vi "ISEG_HVBoard.ProcCases.vi"(0 "i ref in":refnum<vi>, 1 "selector":string, 2 "Data":T1, 3 "call cluster":T2={"Object"="", "Selector"="", "CallType"=enum."synchronous", "Async Object"="", "Async Selector"="", "Data Descriptor"="", "Data"=[], "Error #"=0, "Expire"=0}, 5 "error in (no error)":errorcluster) -> (14 "i ref out":refnum<vi>, 17 "answer cluster":T2={"Object"="", "Selector"="", "CallType"=enum."synchronous", "Async Object"="", "Async Selector"="", "Data Descriptor"="", "Data"=[], "Error #"=0, "Expire"=0}, 19 "error out":errorcluster)   [LabVIEW 2014, in "ISEG_HVBoard.lvlib"]
doc: "This method is called by a process from within the default case in the event loop. The methods of a class that are linked to events will be called from THIS method. Add your code here."
uses:
  ISEG_HVBoard.lvlib
  CSCore/CSSystem/CoreDefs/CoreDefs.call_type.ctl
  CSCore/BaseProcess/BaseProcess.descriptor string definition.ctl
  CSCore/CSSystem/CoreDefs/CoreDefs.rawDataType.ctl
  CSCore/CSApplicationBaseClasses/DeviceBase/DeviceBase.deviceState.ctl
  CSCore/CSSystem/CoreLib/CoreLib.string 2 byte array.vi
  CSCore/CSSystem/CoreLib/CoreLib.byte array 2 double.vi
  CSCore/CSSystem/CoreLib/CoreLib.double 2 byte array.vi
  CSCore/CSSystem/CoreLib/CoreLib.short 2 byte array.vi
  CSCore/CSSystem/CoreLib/CoreLib.byte array 2 short.vi
  CSCore/CSApplicationBaseClasses/DeviceBase/DeviceBase.lvlib
  CSCore/CSSystem/CoreLib/CoreLib.lvlib
  CSCore/BaseProcess/BaseProcess.lvlib
  CSCore/CAEObj/CAEObj.lvlib
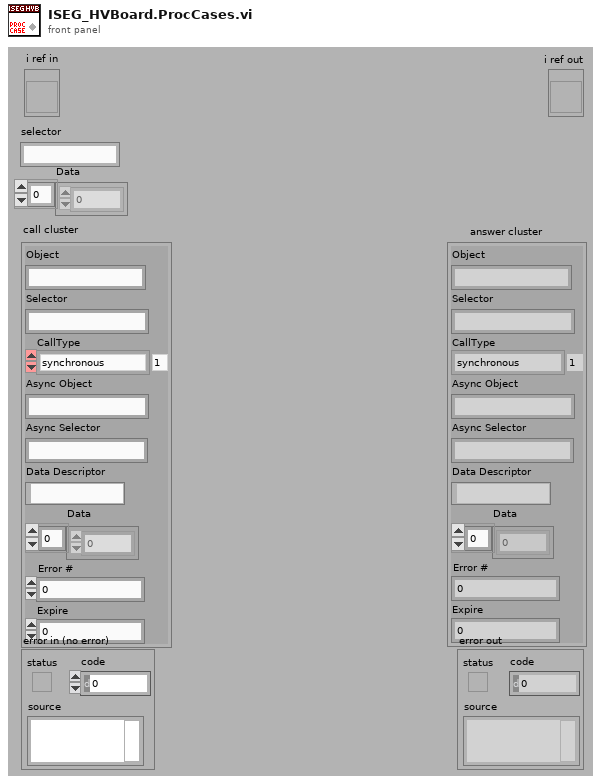
[diagram p1: front panel]
types:
  T1 = typedef "CoreDefs.rawDataType.ctl" = i8[]
  T2 = typedef "CoreDefs.call_type.ctl" = cluster{"Object":string, "Selector":string, "CallType":enum16{"simple", "synchronous", "asynchronous"}, "Async Object":string, "Async Selector":string, "Data Descriptor":T3, "Data":T1, "Error #":i32, "Expire":u32}
  T3 = typedef "BaseProcess.lvlib/BaseProcess.descriptor string definition.ctl" = string
  T4 = typedef "ISEG_HVBoard.lvlib/ISEG_HVBoard.i attribute.ctl" = cluster{"System Name":string, "Board ID":i32, "Prefix":string, "NrOfCh":cluster{"NrOfCh":i16, "DIM Status":T5}, "Status":cluster{"Status":i16, "DIM Status":T5}, "HardwareVLimit":cluster{"HVMax":dbl, "DIM Status":T5}, "BoardTemp":cluster{"Temp":dbl, "DIM Status":T5}, " Emcy":cluster{"Emcy":bool, "DIM Status":T5}}
  T5 = typedef "ISEG_HVBoard.lvlib/ISEG_HVBoard.DIM Status.ctl" = cluster{"no link":bool, "quality":i32, "Time Stamp":timestamp}
  T6 = typedef "DeviceBase.lvlib/DeviceBase.i attribute.ctl" = cluster{"deviceState":i32, "deviceStateID":i32, "deviceID":string, "deviceIDID":i32, "advancedGUIClass":string, "advancedGUIClassID":i32}
  T7 = typedef "DeviceBase.lvlib/DeviceBase.deviceState.ctl" = i16
  T8 = typedef "BaseProcess.lvlib/BaseProcess.i attribute.ctl" = cluster{"EventStatus":string, "EventError":i32, "PresetEvtWatchD":i32, "PresetPdcWatchD":i32, "EventTimeout":i32, "PeriodicInterval":i32, "Interface":string[], "Address":string[], "Special":string[], "PeriodicError":i32, "PeriodicStatus":string, "SuperProc":string, "Descriptors":T9[], "CaseRef":refnum<vi>, "PdcRef":refnum<vi>, "Thread Ref":refnum<vi>, "eventErrorID":i32, "eventStatusID":i32, "periodicErrorID":i32, "periodicStatusID":i32, "pdcCtrID":i32}
  T9 = typedef "BaseProcess.lvlib/BaseProcess.descriptor definition.ctl" = cluster{"selector":string, "descriptor":T3}
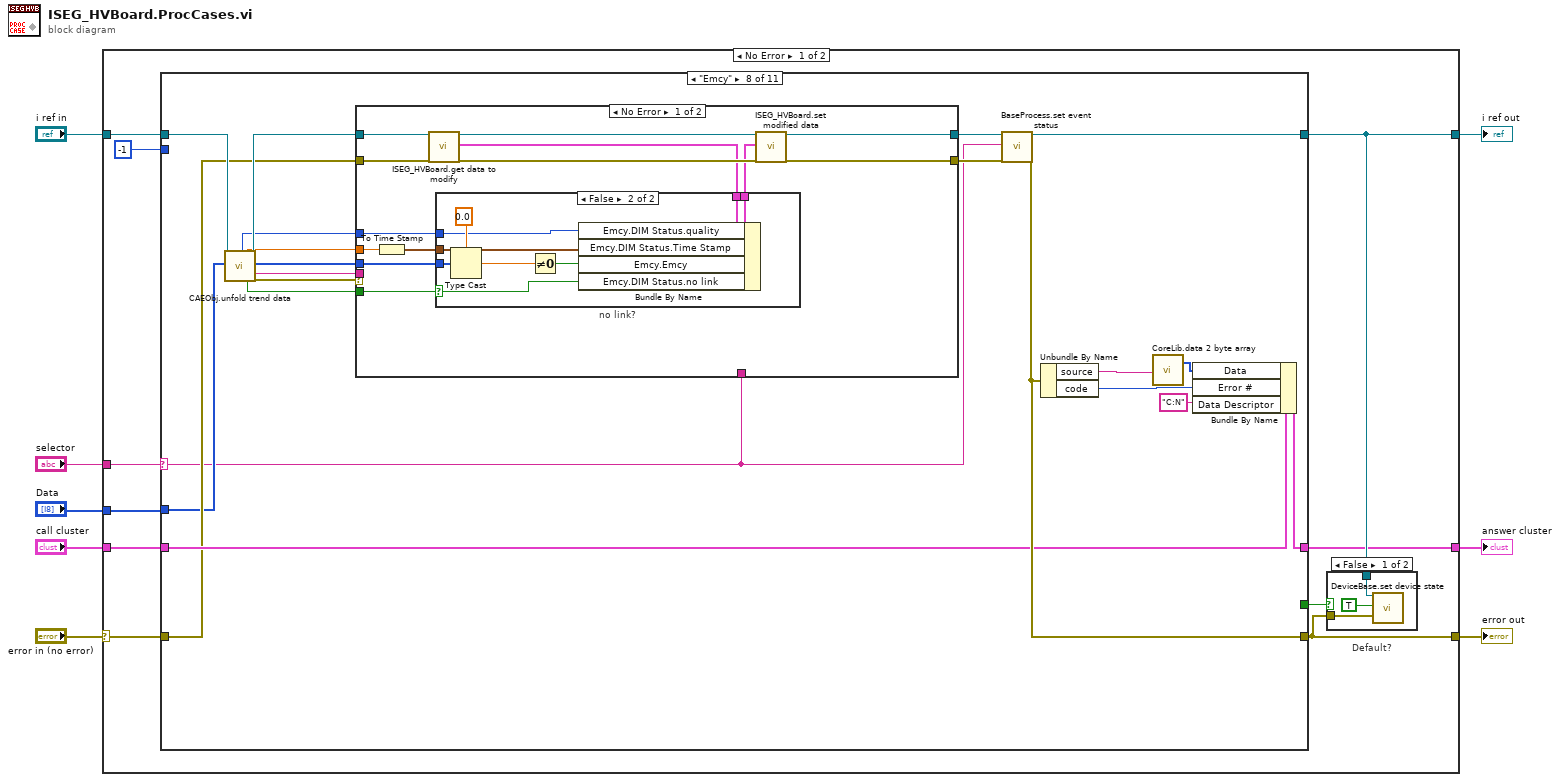
[diagram p0: block diagram]
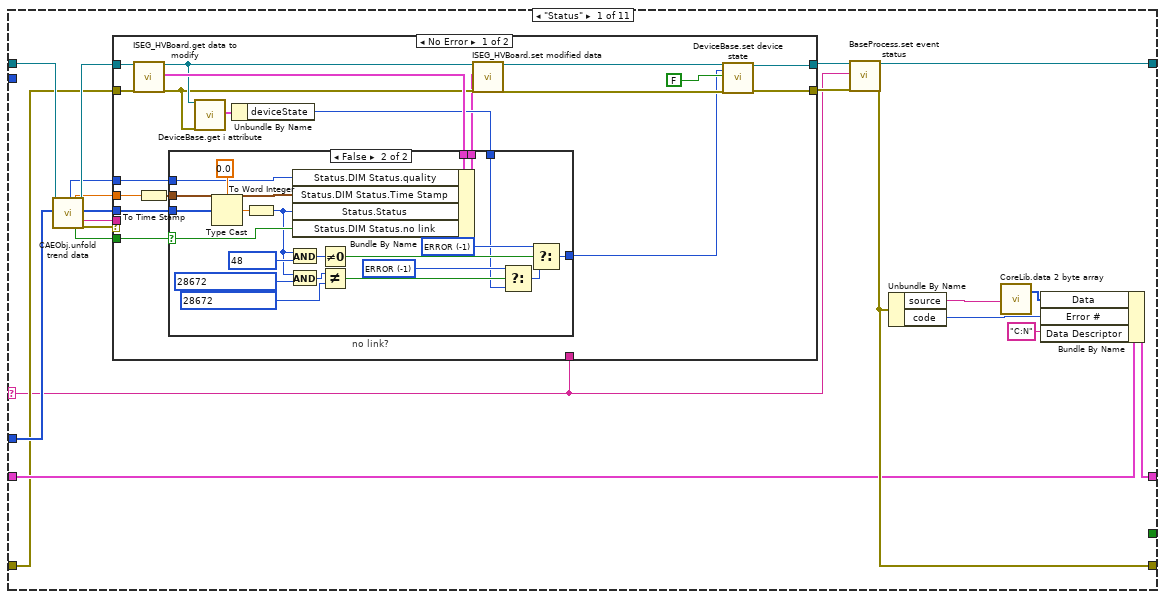
[diagram p3: hidden frame]
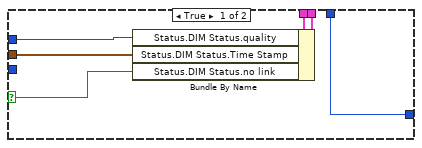
[diagram p4: hidden frame]
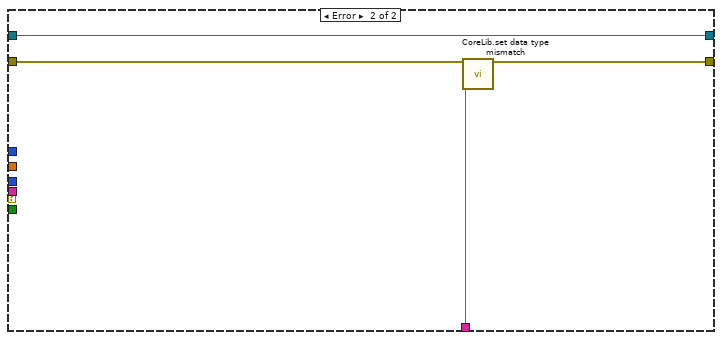
[diagram p5: hidden frame]
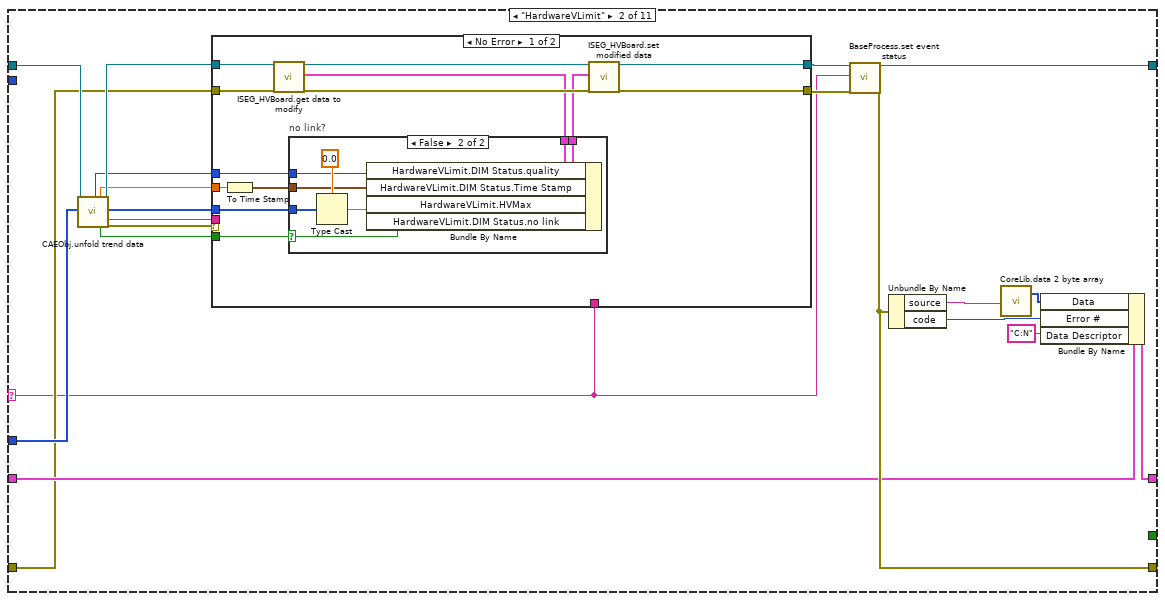
[diagram p6: hidden frame]
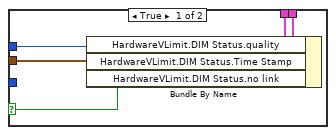
[diagram p7: hidden frame]
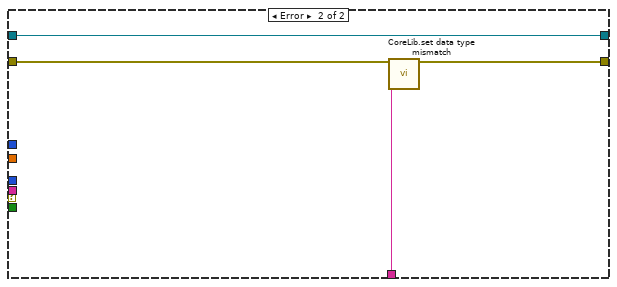
[diagram p8: hidden frame]
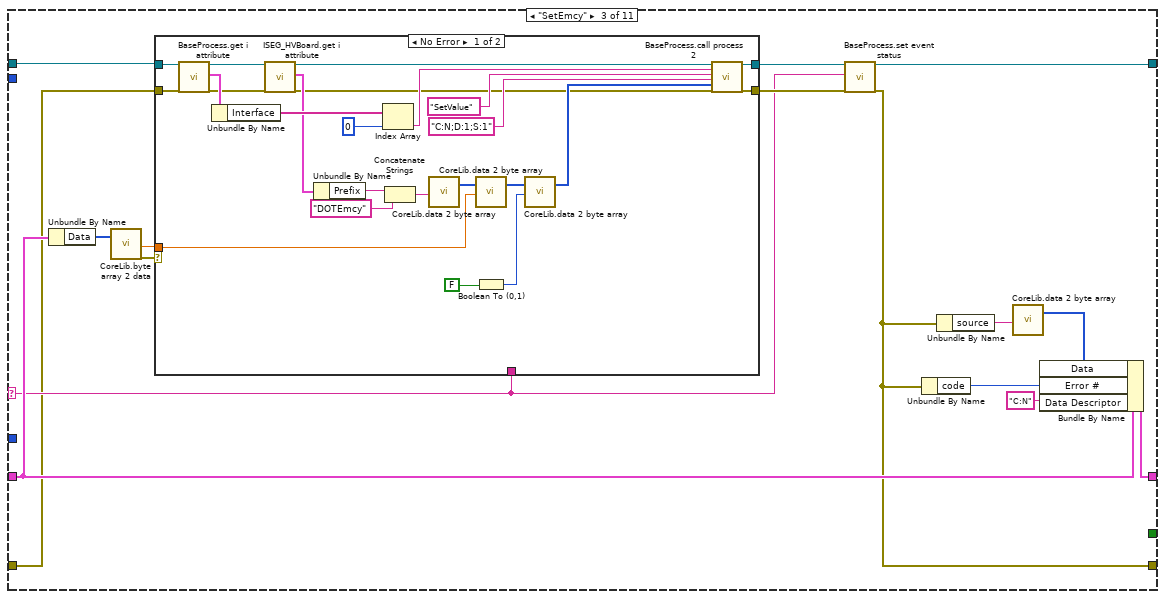
[diagram p9: hidden frame]
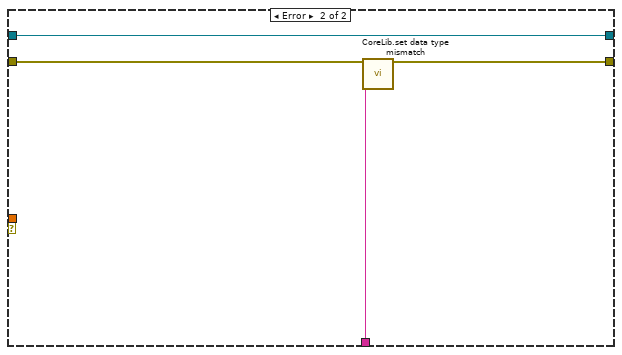
[diagram p10: hidden frame]
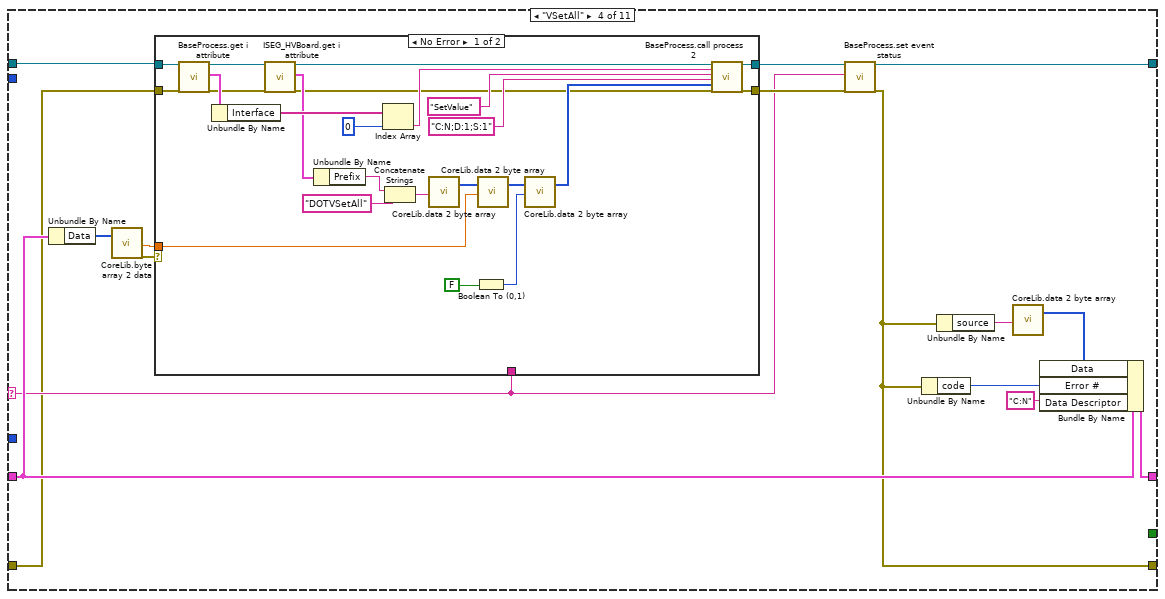
[diagram p11: hidden frame]
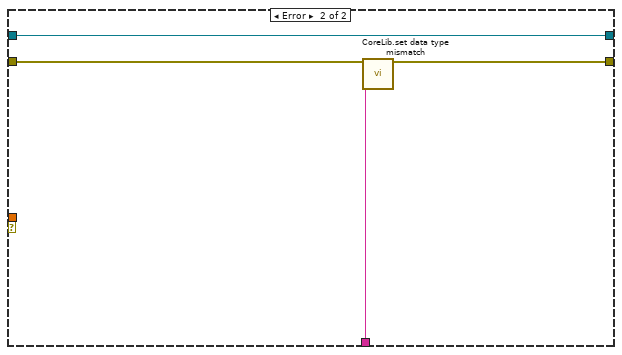
[diagram p12: hidden frame]
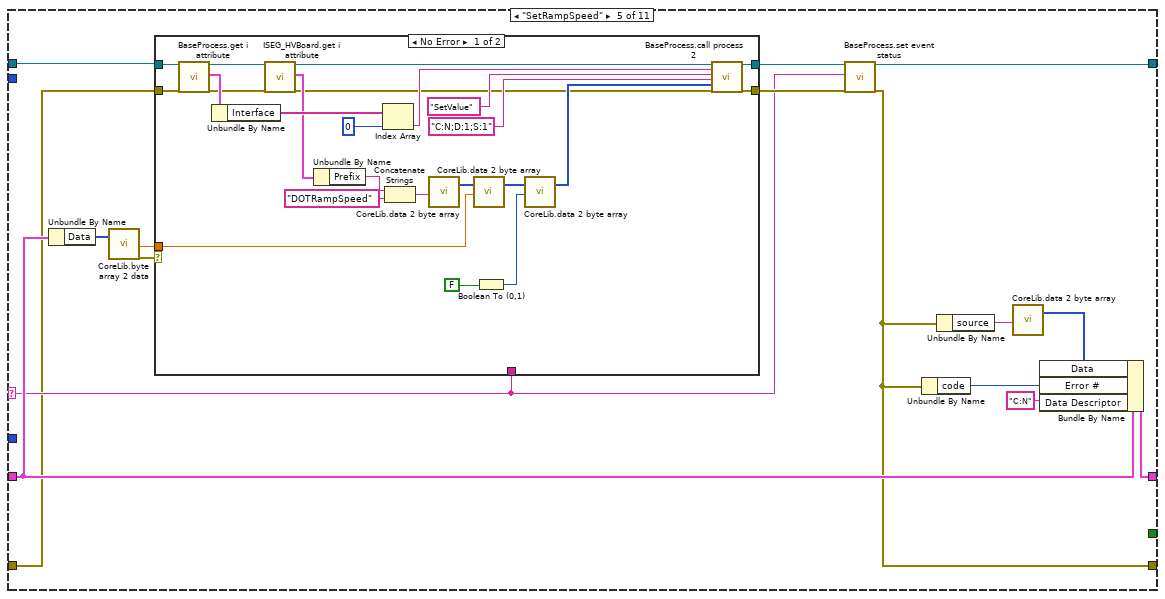
[diagram p13: hidden frame]
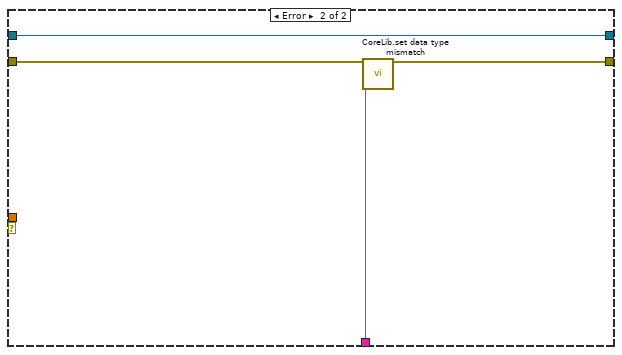
[diagram p14: hidden frame]
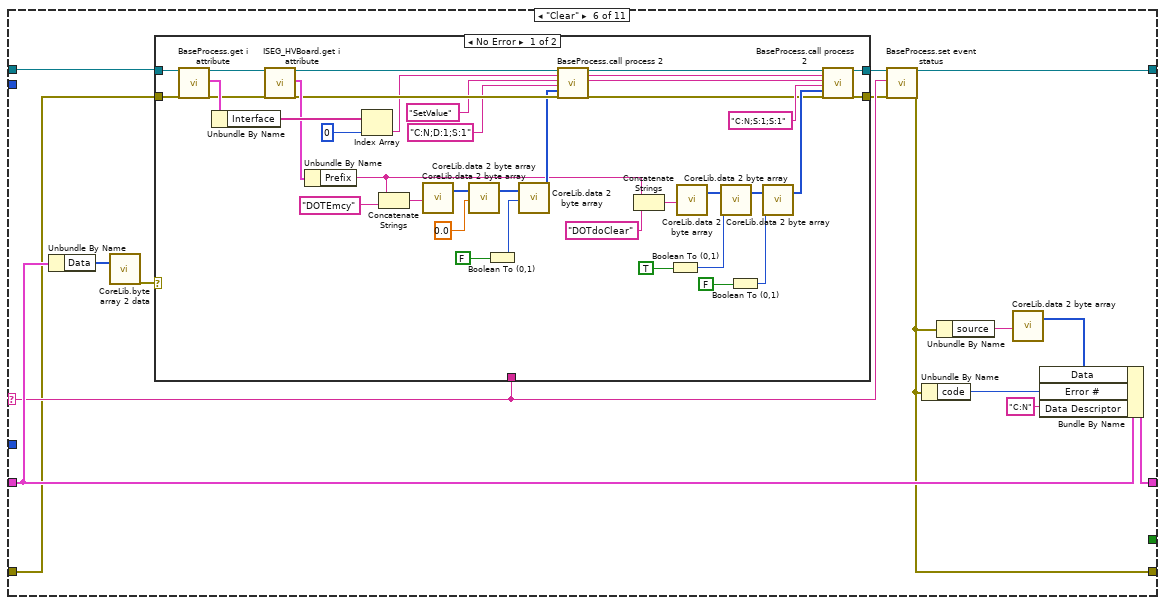
[diagram p15: hidden frame]
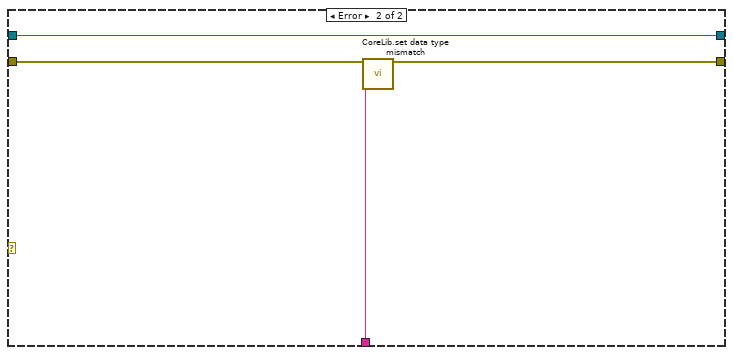
[diagram p16: hidden frame]
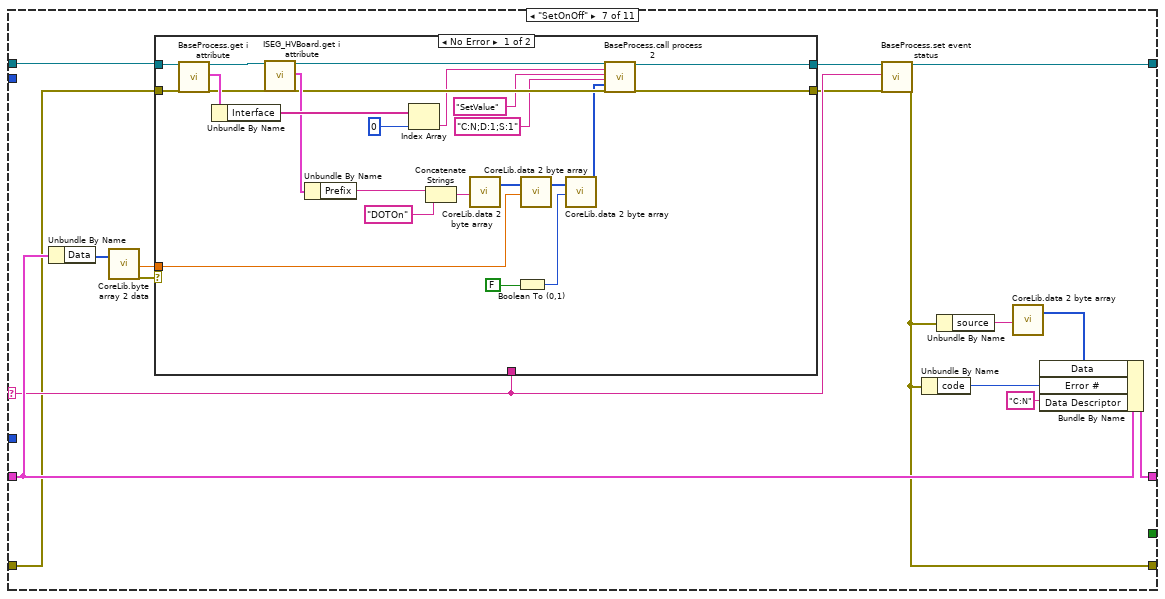
[diagram p17: hidden frame]
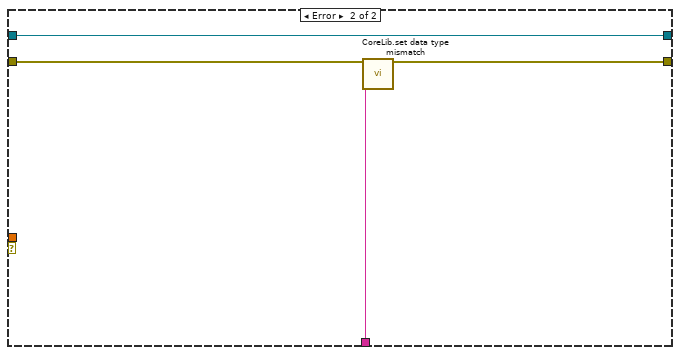
[diagram p18: hidden frame]
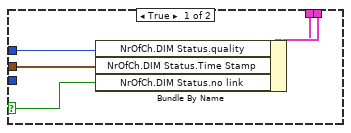
[diagram p19: hidden frame]
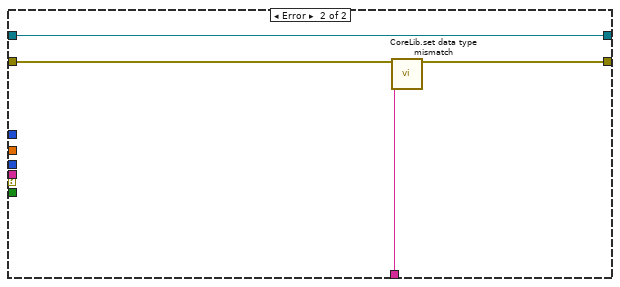
[diagram p20: hidden frame]
diagram:
  n1 = case shown="No Error" "error in (no error)" {
    selector: "error in (no error)" -> [w13 w538]
    tunnel: "selector" -> [w16 _]
    tunnel: [w10 w539] -> w7
    tunnel: "Data" -> [w15 _]
    tunnel: "call cluster" -> [w14 w539]
    tunnel: "i ref in" -> [w18 w540]
    tunnel: [w11 w540] -> w3
    tunnel: [w9 w538] -> w2
    frame No Error {
      n2 = case shown="\"Emcy\"" w16 {
        selector: w16 -> [w22 w93 w150 w194 w238 w282 w338 w375 w429 w479 w532]
        tunnel: w15 -> [w26 w97 _ _ _ _ _ w376 w430 w483 _]
        tunnel: w18 -> [w27 w98 w153 w197 w241 w285 w341 w380 w432 w484 w531]
        tunnel: [w37 w107 w152 w196 w240 w284 w340 w389 w441 w493 w537] -> w11
        tunnel: w14 -> [w36 w106 w151 w195 w239 w283 w339 w388 w440 w492 w533]
        tunnel: [w35 w108 w147 w191 w235 w279 w335 w390 w442 w494 w534] -> w10
        tunnel: w13 -> [w23 w96 w148 w192 w236 w280 w336 w377 w431 w482 w536]
        tunnel: [w38 w109 w149 w193 w237 w281 w337 w391 w443 w495 w535] -> w9
        tunnel: [_ _ _ _ _ _ _ _ _ _ TRUE] -> w12
        tunnel: -1 -> [_ _ _ _ _ _ _ _ _ _ _]
        frame "Status" {
          n3 = call "CAEObj.unfold trend data.vi"("i ref in"=w27, "raw trend data"=w26) -> ("quality"=w31:i32, "timeStamp"=w30:dbl, "no link"=w28:bool, "i ref out"=w34:refnum<vi>, "data"=w33:i8[], "typeDescriptor"=w32:string, "error out"=w29:errorcluster)  [unwired: 9 in, 2 out]
          n4 = case shown="No Error" w29 {
            tunnel: [w47 w92] -> w25
            tunnel: w34 -> [w61 w92]
            tunnel: w23 -> [w60 w91]
            tunnel: [w46 w90] -> w24
            tunnel: w22 -> [_ w89]
            tunnel: w33 -> [w59 _]
            tunnel: w32 -> [_ _]
            tunnel: w31 -> [w57 _]
            tunnel: w30 -> [w55 _]
            tunnel: w28 -> [w54 _]
            frame No Error {
              n5 = call "ISEG_HVBoard.get data to modify.vi"("i ref in"=w61, "error in (no error)"=w60) -> ("i ref out"=w52:refnum<vi>, "i attribute"=w58:T4, "error out"=w51:errorcluster)  [unwired: 14 in, 1 out]
              n6 = To Time Stamp(1:w55) -> (0:w56:timestamp)
              n7 = call "DeviceBase.get i attribute.vi"("i ref in"=w52, "error in (no error)"=w51) -> ("i attribute"=w53:T6)  [unwired: 15 in, 2 out]
              n8 = Unbundle By Name(w53) -> ("deviceState"=w44:i32)
              n9 = case "no link?" shown="False" w54 {
                selector: w54 -> [w63 w81]
                tunnel: [w67 w88] -> w43
                tunnel: w59 -> [_ w87]
                tunnel: w58 -> [w66 w86]
                tunnel: w57 -> [w65 w83]
                tunnel: w56 -> [w64 w82]
                tunnel: [w62 w77] -> w45
                tunnel: w44 -> [w62 w70]
                frame True {
                  n10 = Bundle By Name(cluster=w66, "Status.DIM Status.quality"=w65, "Status.DIM Status.Time Stamp"=w64, "Status.DIM Status.no link"=w63) -> (w67:T4)
                }
                frame False {
                  w72 = T7 -1 items=["ERROR"=-1, "OK"=0, "NOT_OK"=1] ("deviceState")
                  w80 = T7 -1 items=["ERROR"=-1, "OK"=0, "NOT_OK"=1] ("deviceState")
                  n11 = Type Cast(type=0.0, x=w87) -> (*(type *) &x=w85:dbl)
                  n12 = To Word Integer(number=w85) -> (16bit integer=w75:i16)
                  n13 = And(x=w75, y=i16 48) -> (x .and. y?=w79:i16)
                  n14 = And(x=w75, y=i16 28672) -> (x .and. y?=w69:i16)
                  n15 = Bundle By Name(cluster=w86, "Status.DIM Status.quality"=w83, "Status.DIM Status.Time Stamp"=w82, "Status.Status"=w75, "Status.DIM Status.no link"=w81) -> (w88:T4)
                  n16 = Not Equal To 0?(x=w79) -> (x != 0?=w78:bool)
                  n17 = Not Equal?(x=w69, y=i16 28672) -> (x != y?=w73:bool)
                  n18 = Select(t=w72, s=w73, f=w70) -> (s? t:f=w71:i32)
                  n19 = Select(t=w80, s=w78, f=w71) -> (s? t:f=w77:i32)
                }
              }
              n20 = call "ISEG_HVBoard.set modified data.vi"("i ref in"=w52, "i attribute"=w43, "error in (no error)"=w51) -> ("i ref out"=w48:refnum<vi>, "error out"=w49:errorcluster)  [unwired: 15 in]
              n21 = call "DeviceBase.set device state.vi"("i ref in"=w48, "deviceState"=w45, "implicit"=FALSE, "error in (no error)"=w49) -> ("i ref out"=w47:refnum<vi>, "error out"=w46:errorcluster)  [unwired: 13 in, 1 out]
            }
            frame Error {
              n22 = call "CoreLib.set data type mismatch.vi"("error in (no error)"=w91, "error source"=w89) -> ("error out"=w90:errorcluster)  [unwired: 17 in]
            }
          }
          n23 = call "BaseProcess.set event status.vi"("i ref in"=w25, "EventStatus"=w22, "error in (no error)"=w24) -> ("i ref out"=w37:refnum<vi>, "error out"=w38:errorcluster)  [unwired: 14 in, 1 out]
          n24 = Unbundle By Name(w38) -> ("source"=w39:string, "code"=w42:i32)
          n25 = call-poly "CoreLib.data 2 byte array.vi"("string"=w39) -> ("byteArray out"=w41:T1)  [unwired: 18 in]
          n26 = Bundle By Name(cluster=w36, "Data"=w41, "Error #"=w42, "Data Descriptor"="C:N") -> (w35:T2)
        }
        frame "HardwareVLimit" {
          n27 = call "CAEObj.unfold trend data.vi"("i ref in"=w98, "raw trend data"=w97) -> ("quality"=w102:i32, "timeStamp"=w101:dbl, "no link"=w99:bool, "i ref out"=w105:refnum<vi>, "data"=w104:i8[], "typeDescriptor"=w103:string, "error out"=w100:errorcluster)  [unwired: 9 in, 2 out]
          n28 = case shown="No Error" w100 {
            tunnel: [w120 w143] -> w94
            tunnel: w105 -> [w126 w143]
            tunnel: w96 -> [w125 w142]
            tunnel: [w119 w141] -> w95
            tunnel: w93 -> [_ w140]
            tunnel: w104 -> [w121 _]
            tunnel: w103 -> [_ _]
            tunnel: w102 -> [w117 _]
            tunnel: w101 -> [w115 _]
            tunnel: w99 -> [w114 _]
            frame No Error {
              n29 = To Time Stamp(1:w115) -> (0:w116:timestamp)
              n30 = call "ISEG_HVBoard.get data to modify.vi"("i ref in"=w126, "error in (no error)"=w125) -> ("i ref out"=w124:refnum<vi>, "i attribute"=w118:T4, "error out"=w123:errorcluster)  [unwired: 14 in, 1 out]
              n31 = case "no link?" shown="False" w114 {
                selector: w114 -> [w127 w133]
                tunnel: [w131 w139] -> w122
                tunnel: w121 -> [_ w138]
                tunnel: w118 -> [w130 w136]
                tunnel: w117 -> [w129 w135]
                tunnel: w116 -> [w128 w134]
                frame True {
                  n32 = Bundle By Name(cluster=w130, "HardwareVLimit.DIM Status.quality"=w129, "HardwareVLimit.DIM Status.Time Stamp"=w128, "HardwareVLimit.DIM Status.no link"=w127) -> (w131:T4)
                }
                frame False {
                  n33 = Type Cast(type=0.0, x=w138) -> (*(type *) &x=w132:dbl)
                  n34 = Bundle By Name(cluster=w136, "HardwareVLimit.DIM Status.quality"=w135, "HardwareVLimit.DIM Status.Time Stamp"=w134, "HardwareVLimit.HVMax"=w132, "HardwareVLimit.DIM Status.no link"=w133) -> (w139:T4)
                }
              }
              n35 = call "ISEG_HVBoard.set modified data.vi"("i ref in"=w124, "i attribute"=w122, "error in (no error)"=w123) -> ("i ref out"=w120:refnum<vi>, "error out"=w119:errorcluster)  [unwired: 15 in]
            }
            frame Error {
              n36 = call "CoreLib.set data type mismatch.vi"("error in (no error)"=w142, "error source"=w140) -> ("error out"=w141:errorcluster)  [unwired: 17 in]
            }
          }
          n37 = call "BaseProcess.set event status.vi"("i ref in"=w94, "EventStatus"=w93, "error in (no error)"=w95) -> ("i ref out"=w107:refnum<vi>, "error out"=w109:errorcluster)  [unwired: 14 in, 1 out]
          n38 = Unbundle By Name(w109) -> ("source"=w110:string, "code"=w113:i32)
          n39 = call-poly "CoreLib.data 2 byte array.vi"("string"=w110) -> ("byteArray out"=w112:T1)  [unwired: 18 in]
          n40 = Bundle By Name(cluster=w106, "Data"=w112, "Error #"=w113, "Data Descriptor"="C:N") -> (w108:T2)
        }
        frame "SetEmcy" {
          n41 = Unbundle By Name(w151) -> ("Data"=w144:T1)
          n42 = call-poly "CoreLib.byte array 2 data.vi"("byteArray"=w144) -> ("d64"=w146:dbl, "error out"=w145:errorcluster)  [unwired: 16 in, 1 out]
          n43 = case shown="No Error" w145 {
            tunnel: [w183 w187] -> w157
            tunnel: w153 -> [w169 w187]
            tunnel: w148 -> [w181 w186]
            tunnel: [w182 w185] -> w156
            tunnel: w150 -> [_ w184]
            tunnel: w146 -> [w160 _]
            frame No Error {
              n44 = call "BaseProcess.get i attribute.vi"("i ref in"=w169, "error in (no error)"=w181) -> ("i ref out"=w164:refnum<vi>, "i attribute"=w180:T8, "error out"=w166:errorcluster)  [unwired: 15 in]
              n45 = Unbundle By Name(w180) -> ("Interface"=w179:string[])
              n46 = call "ISEG_HVBoard.get i attribute.vi"("i ref in"=w164, "error in (no error)"=w166) -> ("i ref out"=w163:refnum<vi>, "i attribute"=w168:T4, "error out"=w165:errorcluster)  [unwired: 15 in]
              n47 = Unbundle By Name(w168) -> ("Prefix"=w167:string)
              n48 = Index Array(array=w179, index=0) -> (element=w177:string)
              n49 = Concatenate Strings(w167, "DOTEmcy" ("string")) -> (w171:string)
              n50 = call-poly "CoreLib.data 2 byte array.vi"("string"=w171) -> ("byteArray out"=w162:T1)  [unwired: 18 in]
              n51 = call-poly "CoreLib.data 2 byte array.vi"("byteArray"=w162, "f64"=w160) -> ("byteArray out"=w161:T1)  [unwired: 17 in]
              n52 = Boolean To (0,1)(Boolean=FALSE) -> (0, 1=w173:i16)
              n53 = call-poly "CoreLib.data 2 byte array.vi"("byteArray"=w161, "i16"=w173) -> ("byteArray out"=w172:T1)  [unwired: 17 in]
              n54 = call "BaseProcess.call process 2.vi"("i ref in"=w163, "Object"=w177, "Selector"="SetValue", "Data Descriptor"="C:N;D:1;S:1", "Data"=w172, "error in (no error)"=w165) -> ("i ref out"=w183:refnum<vi>, "error out"=w182:errorcluster)  [unwired: 12 in]
            }
            frame Error {
              n55 = call "CoreLib.set data type mismatch.vi"("error in (no error)"=w186, "error source"=w184) -> ("error out"=w185:errorcluster)  [unwired: 17 in]
            }
          }
          n56 = call "BaseProcess.set event status.vi"("i ref in"=w157, "EventStatus"=w150, "error in (no error)"=w156) -> ("i ref out"=w152:refnum<vi>, "error out"=w149:errorcluster)  [unwired: 14 in, 1 out]
          n57 = Unbundle By Name(w149) -> ("code"=w159:i32)
          n58 = Unbundle By Name(w149) -> ("source"=w154:string)
          n59 = call-poly "CoreLib.data 2 byte array.vi"("string"=w154) -> ("byteArray out"=w158:T1)  [unwired: 18 in]
          n60 = Bundle By Name(cluster=w151, "Data"=w158, "Error #"=w159, "Data Descriptor"="C:N") -> (w147:T2)
        }
        frame "VSetAll" {
          n61 = Unbundle By Name(w195) -> ("Data"=w188:T1)
          n62 = call-poly "CoreLib.byte array 2 data.vi"("byteArray"=w188) -> ("d64"=w190:dbl, "error out"=w189:errorcluster)  [unwired: 16 in, 1 out]
          n63 = case shown="No Error" w189 {
            tunnel: [w227 w231] -> w201
            tunnel: w197 -> [w213 w231]
            tunnel: w192 -> [w225 w230]
            tunnel: [w226 w229] -> w200
            tunnel: w194 -> [_ w228]
            tunnel: w190 -> [w204 _]
            frame No Error {
              n64 = call "BaseProcess.get i attribute.vi"("i ref in"=w213, "error in (no error)"=w225) -> ("i ref out"=w208:refnum<vi>, "i attribute"=w224:T8, "error out"=w210:errorcluster)  [unwired: 15 in]
              n65 = Unbundle By Name(w224) -> ("Interface"=w223:string[])
              n66 = call "ISEG_HVBoard.get i attribute.vi"("i ref in"=w208, "error in (no error)"=w210) -> ("i ref out"=w207:refnum<vi>, "i attribute"=w212:T4, "error out"=w209:errorcluster)  [unwired: 15 in]
              n67 = Unbundle By Name(w212) -> ("Prefix"=w211:string)
              n68 = Index Array(array=w223, index=0) -> (element=w221:string)
              n69 = Concatenate Strings(w211, "DOTVSetAll" ("string")) -> (w215:string)
              n70 = call-poly "CoreLib.data 2 byte array.vi"("string"=w215) -> ("byteArray out"=w205:T1)  [unwired: 18 in]
              n71 = Boolean To (0,1)(Boolean=FALSE) -> (0, 1=w217:i16)
              n72 = call-poly "CoreLib.data 2 byte array.vi"("byteArray"=w205, "f64"=w204) -> ("byteArray out"=w206:T1)  [unwired: 17 in]
              n73 = call-poly "CoreLib.data 2 byte array.vi"("byteArray"=w206, "i16"=w217) -> ("byteArray out"=w216:T1)  [unwired: 17 in]
              n74 = call "BaseProcess.call process 2.vi"("i ref in"=w207, "Object"=w221, "Selector"="SetValue", "Data Descriptor"="C:N;D:1;S:1", "Data"=w216, "error in (no error)"=w209) -> ("i ref out"=w227:refnum<vi>, "error out"=w226:errorcluster)  [unwired: 12 in]
            }
            frame Error {
              n75 = call "CoreLib.set data type mismatch.vi"("error in (no error)"=w230, "error source"=w228) -> ("error out"=w229:errorcluster)  [unwired: 17 in]
            }
          }
          n76 = call "BaseProcess.set event status.vi"("i ref in"=w201, "EventStatus"=w194, "error in (no error)"=w200) -> ("i ref out"=w196:refnum<vi>, "error out"=w193:errorcluster)  [unwired: 14 in, 1 out]
          n77 = Unbundle By Name(w193) -> ("code"=w203:i32)
          n78 = Unbundle By Name(w193) -> ("source"=w198:string)
          n79 = call-poly "CoreLib.data 2 byte array.vi"("string"=w198) -> ("byteArray out"=w202:T1)  [unwired: 18 in]
          n80 = Bundle By Name(cluster=w195, "Data"=w202, "Error #"=w203, "Data Descriptor"="C:N") -> (w191:T2)
        }
        frame "SetRampSpeed" {
          n81 = Unbundle By Name(w239) -> ("Data"=w232:T1)
          n82 = call-poly "CoreLib.byte array 2 data.vi"("byteArray"=w232) -> ("d64"=w234:dbl, "error out"=w233:errorcluster)  [unwired: 16 in, 1 out]
          n83 = case shown="No Error" w233 {
            tunnel: [w271 w275] -> w245
            tunnel: w241 -> [w258 w275]
            tunnel: w236 -> [w269 w274]
            tunnel: [w270 w273] -> w244
            tunnel: w238 -> [_ w272]
            tunnel: w234 -> [w248 _]
            frame No Error {
              n84 = call "BaseProcess.get i attribute.vi"("i ref in"=w258, "error in (no error)"=w269) -> ("i ref out"=w253:refnum<vi>, "i attribute"=w268:T8, "error out"=w255:errorcluster)  [unwired: 15 in]
              n85 = Unbundle By Name(w268) -> ("Interface"=w267:string[])
              n86 = call "ISEG_HVBoard.get i attribute.vi"("i ref in"=w253, "error in (no error)"=w255) -> ("i ref out"=w252:refnum<vi>, "i attribute"=w257:T4, "error out"=w254:errorcluster)  [unwired: 15 in]
              n87 = Unbundle By Name(w257) -> ("Prefix"=w256:string)
              n88 = Index Array(array=w267, index=0) -> (element=w265:string)
              n89 = Concatenate Strings(w256, "DOTRampSpeed" ("string")) -> (w259:string)
              n90 = call-poly "CoreLib.data 2 byte array.vi"("string"=w259) -> ("byteArray out"=w250:T1)  [unwired: 18 in]
              n91 = call-poly "CoreLib.data 2 byte array.vi"("byteArray"=w250, "f64"=w248) -> ("byteArray out"=w249:T1)  [unwired: 17 in]
              n92 = Boolean To (0,1)(Boolean=FALSE) -> (0, 1=w261:i16)
              n93 = call-poly "CoreLib.data 2 byte array.vi"("byteArray"=w249, "i16"=w261) -> ("byteArray out"=w260:T1)  [unwired: 17 in]
              n94 = call "BaseProcess.call process 2.vi"("i ref in"=w252, "Object"=w265, "Selector"="SetValue", "Data Descriptor"="C:N;D:1;S:1", "Data"=w260, "error in (no error)"=w254) -> ("i ref out"=w271:refnum<vi>, "error out"=w270:errorcluster)  [unwired: 12 in]
            }
            frame Error {
              n95 = call "CoreLib.set data type mismatch.vi"("error in (no error)"=w274, "error source"=w272) -> ("error out"=w273:errorcluster)  [unwired: 17 in]
            }
          }
          n96 = call "BaseProcess.set event status.vi"("i ref in"=w245, "EventStatus"=w238, "error in (no error)"=w244) -> ("i ref out"=w240:refnum<vi>, "error out"=w237:errorcluster)  [unwired: 14 in, 1 out]
          n97 = Unbundle By Name(w237) -> ("code"=w247:i32)
          n98 = Unbundle By Name(w237) -> ("source"=w242:string)
          n99 = call-poly "CoreLib.data 2 byte array.vi"("string"=w242) -> ("byteArray out"=w246:T1)  [unwired: 18 in]
          n100 = Bundle By Name(cluster=w239, "Data"=w246, "Error #"=w247, "Data Descriptor"="C:N") -> (w235:T2)
        }
        frame "Clear" {
          n101 = Unbundle By Name(w283) -> ("Data"=w276:T1)
          n102 = call-poly "CoreLib.byte array 2 data.vi"("byteArray"=w276) -> ("error out"=w277:errorcluster)  [unwired: 16 in, 2 out]
          n103 = case shown="No Error" w277 {
            tunnel: [w298 w330] -> w288
            tunnel: w285 -> [w323 w330]
            tunnel: w280 -> [w326 w329]
            tunnel: w282 -> [_ w328]
            tunnel: [w297 w327] -> w278
            frame No Error {
              w294 = "SetValue" ("Selector")
              n104 = call "BaseProcess.get i attribute.vi"("i ref in"=w323, "error in (no error)"=w326) -> ("i ref out"=w319:refnum<vi>, "i attribute"=w325:T8, "error out"=w321:errorcluster)  [unwired: 15 in]
              n105 = Unbundle By Name(w325) -> ("Interface"=w324:string[])
              n106 = call "ISEG_HVBoard.get i attribute.vi"("i ref in"=w319, "error in (no error)"=w321) -> ("i ref out"=w318:refnum<vi>, "i attribute"=w322:T4, "error out"=w320:errorcluster)  [unwired: 15 in]
              n107 = Unbundle By Name(w322) -> ("Prefix"=w296:string)
              n108 = Index Array(array=w324, index=0) -> (element=w295:string)
              n109 = Concatenate Strings(w296, "DOTEmcy" ("string")) -> (w312:string)
              n110 = call-poly "CoreLib.data 2 byte array.vi"("string"=w312) -> ("byteArray out"=w293:T1)  [unwired: 18 in]
              n111 = call-poly "CoreLib.data 2 byte array.vi"("byteArray"=w293, "f64"=0.0) -> ("byteArray out"=w292:T1)  [unwired: 17 in]
              n112 = Boolean To (0,1)(Boolean=FALSE) -> (0, 1=w314:i16)
              n113 = call-poly "CoreLib.data 2 byte array.vi"("byteArray"=w292, "i16"=w314) -> ("byteArray out"=w313:T1)  [unwired: 17 in]
              n114 = call "BaseProcess.call process 2.vi"("i ref in"=w318, "Object"=w295, "Selector"=w294, "Data Descriptor"="C:N;D:1;S:1", "Data"=w313, "error in (no error)"=w320) -> ("i ref out"=w300:refnum<vi>, "error out"=w299:errorcluster)  [unwired: 12 in]
              n115 = Concatenate Strings(w296, "DOTdoClear" ("string")) -> (w308:string)
              n116 = Boolean To (0,1)(Boolean=TRUE) -> (0, 1=w305:i16)
              n117 = call-poly "CoreLib.data 2 byte array.vi"("string"=w308) -> ("byteArray out"=w304:T1)  [unwired: 18 in]
              n118 = call-poly "CoreLib.data 2 byte array.vi"("byteArray"=w304, "i16"=w305) -> ("byteArray out"=w303:T1)  [unwired: 17 in]
              n119 = Boolean To (0,1)(Boolean=FALSE) -> (0, 1=w309:i16)
              n120 = call-poly "CoreLib.data 2 byte array.vi"("byteArray"=w303, "i16"=w309) -> ("byteArray out"=w301:T1)  [unwired: 17 in]
              n121 = call "BaseProcess.call process 2.vi"("i ref in"=w300, "Object"=w295, "Selector"=w294, "Data Descriptor"="C:N;S:1;S:1", "Data"=w301, "error in (no error)"=w299) -> ("i ref out"=w298:refnum<vi>, "error out"=w297:errorcluster)  [unwired: 12 in]
            }
            frame Error {
              n122 = call "CoreLib.set data type mismatch.vi"("error in (no error)"=w329, "error source"=w328) -> ("error out"=w327:errorcluster)  [unwired: 17 in]
            }
          }
          n123 = call "BaseProcess.set event status.vi"("i ref in"=w288, "EventStatus"=w282, "error in (no error)"=w278) -> ("i ref out"=w284:refnum<vi>, "error out"=w281:errorcluster)  [unwired: 14 in, 1 out]
          n124 = Unbundle By Name(w281) -> ("code"=w290:i32)
          n125 = Unbundle By Name(w281) -> ("source"=w286:string)
          n126 = call-poly "CoreLib.data 2 byte array.vi"("string"=w286) -> ("byteArray out"=w289:T1)  [unwired: 18 in]
          n127 = Bundle By Name(cluster=w283, "Data"=w289, "Error #"=w290, "Data Descriptor"="C:N") -> (w279:T2)
        }
        frame "SetOnOff" {
          n128 = Unbundle By Name(w339) -> ("Data"=w331:T1)
          n129 = call-poly "CoreLib.byte array 2 data.vi"("byteArray"=w331) -> ("d64"=w333:dbl, "error out"=w332:errorcluster)  [unwired: 16 in, 1 out]
          n130 = case shown="No Error" w332 {
            tunnel: [w359 w374] -> w344
            tunnel: w341 -> [w367 w374]
            tunnel: w336 -> [w370 w373]
            tunnel: w338 -> [_ w372]
            tunnel: [w360 w371] -> w334
            tunnel: w333 -> [w347 _]
            frame No Error {
              n131 = call "BaseProcess.get i attribute.vi"("i ref in"=w367, "error in (no error)"=w370) -> ("i ref out"=w363:refnum<vi>, "i attribute"=w369:T8, "error out"=w365:errorcluster)  [unwired: 15 in]
              n132 = Unbundle By Name(w369) -> ("Interface"=w368:string[])
              n133 = call "ISEG_HVBoard.get i attribute.vi"("i ref in"=w363, "error in (no error)"=w365) -> ("i ref out"=w362:refnum<vi>, "i attribute"=w366:T4, "error out"=w364:errorcluster)  [unwired: 15 in]
              n134 = Unbundle By Name(w366) -> ("Prefix"=w361:string)
              n135 = Index Array(array=w368, index=0) -> (element=w351:string)
              n136 = Concatenate Strings(w361, "DOTOn" ("string")) -> (w353:string)
              n137 = call-poly "CoreLib.data 2 byte array.vi"("string"=w353) -> ("byteArray out"=w348:T1)  [unwired: 18 in]
              n138 = Boolean To (0,1)(Boolean=FALSE) -> (0, 1=w355:i16)
              n139 = call-poly "CoreLib.data 2 byte array.vi"("byteArray"=w348, "f64"=w347) -> ("byteArray out"=w349:T1)  [unwired: 17 in]
              n140 = call-poly "CoreLib.data 2 byte array.vi"("byteArray"=w349, "i16"=w355) -> ("byteArray out"=w354:T1)  [unwired: 17 in]
              n141 = call "BaseProcess.call process 2.vi"("i ref in"=w362, "Object"=w351, "Selector"="SetValue", "Data Descriptor"="C:N;D:1;S:1", "Data"=w354, "error in (no error)"=w364) -> ("i ref out"=w359:refnum<vi>, "error out"=w360:errorcluster)  [unwired: 12 in]
            }
            frame Error {
              n142 = call "CoreLib.set data type mismatch.vi"("error in (no error)"=w373, "error source"=w372) -> ("error out"=w371:errorcluster)  [unwired: 17 in]
            }
          }
          n143 = call "BaseProcess.set event status.vi"("i ref in"=w344, "EventStatus"=w338, "error in (no error)"=w334) -> ("i ref out"=w340:refnum<vi>, "error out"=w337:errorcluster)  [unwired: 14 in, 1 out]
          n144 = Unbundle By Name(w337) -> ("code"=w346:i32)
          n145 = Unbundle By Name(w337) -> ("source"=w342:string)
          n146 = call-poly "CoreLib.data 2 byte array.vi"("string"=w342) -> ("byteArray out"=w345:T1)  [unwired: 18 in]
          n147 = Bundle By Name(cluster=w339, "Data"=w345, "Error #"=w346, "Data Descriptor"="C:N") -> (w335:T2)
        }
        frame "Emcy" {
          n148 = call "CAEObj.unfold trend data.vi"("i ref in"=w380, "raw trend data"=w376) -> ("quality"=w383:i32, "timeStamp"=w382:dbl, "no link"=w381:bool, "i ref out"=w387:refnum<vi>, "data"=w386:i8[], "typeDescriptor"=w385:string, "error out"=w384:errorcluster)  [unwired: 9 in, 2 out]
          n149 = case shown="No Error" w384 {
            tunnel: [w401 w426] -> w379
            tunnel: w387 -> [w408 w426]
            tunnel: w377 -> [w407 w425]
            tunnel: [w400 w424] -> w378
            tunnel: w375 -> [_ w423]
            tunnel: w386 -> [w403 _]
            tunnel: w385 -> [_ _]
            tunnel: w383 -> [w399 _]
            tunnel: w382 -> [w398 _]
            tunnel: w381 -> [w396 _]
            frame No Error {
              n150 = To Time Stamp(1:w398) -> (0:w397:timestamp)
              n151 = call "ISEG_HVBoard.get data to modify.vi"("i ref in"=w408, "error in (no error)"=w407) -> ("i ref out"=w406:refnum<vi>, "i attribute"=w402:T4, "error out"=w405:errorcluster)  [unwired: 14 in, 1 out]
              n152 = case "no link?" shown="False" w396 {
                selector: w396 -> [w409 w416]
                tunnel: [w413 w422] -> w404
                tunnel: w403 -> [_ w421]
                tunnel: w402 -> [w412 w420]
                tunnel: w399 -> [w411 w418]
                tunnel: w397 -> [w410 w417]
                frame True {
                  n153 = Bundle By Name(cluster=w412, "NrOfCh.DIM Status.quality"=w411, "NrOfCh.DIM Status.Time Stamp"=w410, "NrOfCh.DIM Status.no link"=w409) -> (w413:T4)
                }
                frame False {
                  n154 = Type Cast(type=0.0, x=w421) -> (*(type *) &x=w414:dbl)
                  n155 = Not Equal To 0?(x=w414) -> (x != 0?=w415:bool)
                  n156 = Bundle By Name(cluster=w420, "Emcy.DIM Status.quality"=w418, "Emcy.DIM Status.Time Stamp"=w417, "Emcy.Emcy"=w415, "Emcy.DIM Status.no link"=w416) -> (w422:T4)
                }
              }
              n157 = call "ISEG_HVBoard.set modified data.vi"("i ref in"=w406, "i attribute"=w404, "error in (no error)"=w405) -> ("i ref out"=w401:refnum<vi>, "error out"=w400:errorcluster)  [unwired: 15 in]
            }
            frame Error {
              n158 = call "CoreLib.set data type mismatch.vi"("error in (no error)"=w425, "error source"=w423) -> ("error out"=w424:errorcluster)  [unwired: 17 in]
            }
          }
          n159 = call "BaseProcess.set event status.vi"("i ref in"=w379, "EventStatus"=w375, "error in (no error)"=w378) -> ("i ref out"=w389:refnum<vi>, "error out"=w391:errorcluster)  [unwired: 14 in, 1 out]
          n160 = Unbundle By Name(w391) -> ("source"=w392:string, "code"=w395:i32)
          n161 = call-poly "CoreLib.data 2 byte array.vi"("string"=w392) -> ("byteArray out"=w394:T1)  [unwired: 18 in]
          n162 = Bundle By Name(cluster=w388, "Data"=w394, "Error #"=w395, "Data Descriptor"="C:N") -> (w390:T2)
        }
        frame "NrOfCh" {
          n163 = call "CAEObj.unfold trend data.vi"("i ref in"=w432, "raw trend data"=w430) -> ("quality"=w435:i32, "timeStamp"=w434:dbl, "no link"=w433:bool, "i ref out"=w439:refnum<vi>, "data"=w438:i8[], "typeDescriptor"=w437:string, "error out"=w436:errorcluster)  [unwired: 9 in, 2 out]
          n164 = case shown="No Error" w436 {
            tunnel: [w453 w478] -> w427
            tunnel: w439 -> [w460 w478]
            tunnel: w431 -> [w459 w477]
            tunnel: [w452 w476] -> w428
            tunnel: w429 -> [_ w475]
            tunnel: w438 -> [w455 _]
            tunnel: w437 -> [_ _]
            tunnel: w435 -> [w451 _]
            tunnel: w434 -> [w450 _]
            tunnel: w433 -> [w448 _]
            frame No Error {
              n165 = To Time Stamp(1:w450) -> (0:w449:timestamp)
              n166 = call "ISEG_HVBoard.get data to modify.vi"("i ref in"=w460, "error in (no error)"=w459) -> ("i ref out"=w458:refnum<vi>, "i attribute"=w454:T4, "error out"=w457:errorcluster)  [unwired: 14 in, 1 out]
              n167 = case "no link?" shown="False" w448 {
                selector: w448 -> [w461 w466]
                tunnel: [w465 w474] -> w456
                tunnel: w455 -> [_ w473]
                tunnel: w454 -> [w464 w472]
                tunnel: w451 -> [w463 w468]
                tunnel: w449 -> [w462 w467]
                frame True {
                  n168 = Bundle By Name(cluster=w464, "NrOfCh.DIM Status.quality"=w463, "NrOfCh.DIM Status.Time Stamp"=w462, "NrOfCh.DIM Status.no link"=w461) -> (w465:T4)
                }
                frame False {
                  n169 = Type Cast(type=0.0, x=w473) -> (*(type *) &x=w471:dbl)
                  n170 = To Word Integer(number=w471) -> (16bit integer=w469:i16)
                  n171 = Bundle By Name(cluster=w472, "NrOfCh.DIM Status.quality"=w468, "NrOfCh.DIM Status.Time Stamp"=w467, "NrOfCh.NrOfCh"=w469, "NrOfCh.DIM Status.no link"=w466) -> (w474:T4)
                }
              }
              n172 = call "ISEG_HVBoard.set modified data.vi"("i ref in"=w458, "i attribute"=w456, "error in (no error)"=w457) -> ("i ref out"=w453:refnum<vi>, "error out"=w452:errorcluster)  [unwired: 15 in]
            }
            frame Error {
              n173 = call "CoreLib.set data type mismatch.vi"("error in (no error)"=w477, "error source"=w475) -> ("error out"=w476:errorcluster)  [unwired: 17 in]
            }
          }
          n174 = call "BaseProcess.set event status.vi"("i ref in"=w427, "EventStatus"=w429, "error in (no error)"=w428) -> ("i ref out"=w441:refnum<vi>, "error out"=w443:errorcluster)  [unwired: 14 in, 1 out]
          n175 = Unbundle By Name(w443) -> ("source"=w444:string, "code"=w447:i32)
          n176 = call-poly "CoreLib.data 2 byte array.vi"("string"=w444) -> ("byteArray out"=w446:T1)  [unwired: 18 in]
          n177 = Bundle By Name(cluster=w440, "Data"=w446, "Error #"=w447, "Data Descriptor"="C:N") -> (w442:T2)
        }
        frame "BoardTemp" {
          n178 = call "CAEObj.unfold trend data.vi"("i ref in"=w484, "raw trend data"=w483) -> ("quality"=w487:i32, "timeStamp"=w486:dbl, "no link"=w485:bool, "i ref out"=w491:refnum<vi>, "data"=w490:i8[], "typeDescriptor"=w489:string, "error out"=w488:errorcluster)  [unwired: 9 in, 2 out]
          n179 = case shown="No Error" w488 {
            tunnel: [w506 w529] -> w480
            tunnel: w491 -> [w512 w529]
            tunnel: w482 -> [w511 w528]
            tunnel: [w505 w527] -> w481
            tunnel: w479 -> [_ w526]
            tunnel: w490 -> [w507 _]
            tunnel: w489 -> [_ _]
            tunnel: w487 -> [w503 _]
            tunnel: w486 -> [w501 _]
            tunnel: w485 -> [w500 _]
            frame No Error {
              n180 = To Time Stamp(1:w501) -> (0:w502:timestamp)
              n181 = call "ISEG_HVBoard.get data to modify.vi"("i ref in"=w512, "error in (no error)"=w511) -> ("i ref out"=w510:refnum<vi>, "i attribute"=w504:T4, "error out"=w509:errorcluster)  [unwired: 14 in, 1 out]
              n182 = case "no link?" shown="True" w500 {
                selector: w500 -> [w513 w520]
                tunnel: [w517 w525] -> w508
                tunnel: w507 -> [_ w524]
                tunnel: w504 -> [w516 w523]
                tunnel: w503 -> [w515 w522]
                tunnel: w502 -> [w514 w521]
                frame True {
                  n183 = Bundle By Name(cluster=w516, "BoardTemp.DIM Status.quality"=w515, "BoardTemp.DIM Status.Time Stamp"=w514, "BoardTemp.DIM Status.no link"=w513) -> (w517:T4)
                }
                frame False {
                  n184 = Type Cast(type=0.0, x=w524) -> (*(type *) &x=w519:dbl)
                  n185 = Bundle By Name(cluster=w523, "BoardTemp.DIM Status.quality"=w522, "BoardTemp.DIM Status.Time Stamp"=w521, "BoardTemp.Temp"=w519, "BoardTemp.DIM Status.no link"=w520) -> (w525:T4)
                }
              }
              n186 = call "ISEG_HVBoard.set modified data.vi"("i ref in"=w510, "i attribute"=w508, "error in (no error)"=w509) -> ("i ref out"=w506:refnum<vi>, "error out"=w505:errorcluster)  [unwired: 15 in]
            }
            frame Error {
              n187 = call "CoreLib.set data type mismatch.vi"("error in (no error)"=w528, "error source"=w526) -> ("error out"=w527:errorcluster)  [unwired: 17 in]
            }
          }
          n188 = call "BaseProcess.set event status.vi"("i ref in"=w480, "EventStatus"=w479, "error in (no error)"=w481) -> ("i ref out"=w493:refnum<vi>, "error out"=w495:errorcluster)  [unwired: 14 in, 1 out]
          n189 = Unbundle By Name(w495) -> ("source"=w496:string, "code"=w499:i32)
          n190 = call-poly "CoreLib.data 2 byte array.vi"("string"=w496) -> ("byteArray out"=w498:T1)  [unwired: 18 in]
          n191 = Bundle By Name(cluster=w492, "Data"=w498, "Error #"=w499, "Data Descriptor"="C:N") -> (w494:T2)
        }
        frame Default {
          n192 = call "DeviceBase.ProcCases.vi"("i ref in"=w531, "selector"=w532, "call cluster"=w533, "error in (no error)"=w536) -> ("i ref out"=w537:refnum<vi>, "answer cluster"=w534:T2, "error out"=w535:errorcluster)  [unwired: 13 in]
        }
      }
      n193 = case "Default?" shown="False" w12 {
        tunnel: w9 -> [w20 _]
        tunnel: w11 -> [w19 _]
        frame False {
          n194 = call "DeviceBase.set device state.vi"("i ref in"=w19, "implicit"=TRUE, "device error"=w20) -> ()  [unwired: 14 in, 3 out]
        }
        frame True {
        }
      }
    }
    frame Error {
    }
  }
  "answer cluster" <- w7
  "i ref out" <- w3
  "error out" <- w2
